vi "Stoerungen (65-128)- Allgemein.vi"(8 "Fehler (Eingang)":errorcluster caption="Fehler (Eingang, kein Fehler)") -> (0 "Fehler (Ausgang)":errorcluster)   [LabVIEW 2020, in "Stoermeldungen.lvlib"]
uses:
  Stoermeldungen.lvlib
  Stoerungen 65-128.ctl
  Seiten/Anlagengrenzwerte/Anlagen-Parameternamen.ctl
  Aktion Anlagengrenzen pruefen.ctl
  FGV Stoerungen Aktionen.ctl
  Verwaltung/FGV IN Aktionen.ctl
  Verwaltung/FGV OUT Aktionen.ctl
  Allgemein/FGV Analysator aktiv.ctl
  Konfig-Dateien/FGV Betriebsdaten Aktionen.ctl
  Allgemein/FGV Zustaende Aktionen.ctl
  Funktionstasten/Zustaende.ctl
  Stickstoff Befuellung/Aktionen Stockstoff Befuellung.ctl
  Seiten/Anlagengrenzwerte/Anlagengrenzwerte.lvlib
  Stickstoff Befuellung/Stickstoff Befuellung.lvlib
  Verwaltung/Verwaltung - cRIO.lvlib
  Allgemein/Allgemein.lvlib
  Konfig-Dateien/Konfig-Dateien.lvlib
  Funktionstasten/Funktionstasten.lvlib
  Externe Stickstoff Befuellung/Externe Stickstoff Befuellung.lvlib
  Externe Stickstoff Befuellung/Aktionen Externe Stockstoff Befuellung.ctl
panel:
  # "Störmeldungen:\n\nAllgemein (65-128)"
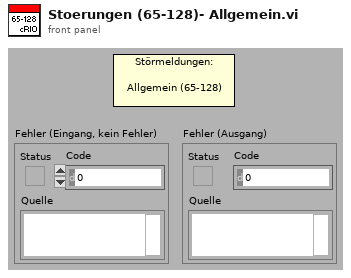
[diagram p1: front panel]
types:
  T1 = typedef "Funktionstasten.lvlib/Zustaende.ctl" = enum16{"Standby", "Pause", "Eco", "Messen", "Kalibrieren", "Spülen Filter", "Spülen Leitung", "Umgebungsluft", "0-Gas", "Cal-Gas", "CG zu PNS", "-------------", "Init 1", "Init 2", "Init 3", "Init 4", "Messen vorbereiten", "Messen durchführen", "Exit"}
  T2 = typedef "Allgemein.lvlib/FGV Zustaende Aktionen.ctl" = enum16{"lesen", "Zustand PC", "Zustand cRIO", "Bildnummer", "Samplepoint", "Sysloglevel"}
  T3 = typedef "Konfig-Dateien.lvlib/FGV Betriebsdaten Aktionen.ctl" = enum16{"lesen", "Anlagengrenzw.", "PID Param.", "Sonstige", "Sensor Para."}
  T4 = typedef "Allgemein.lvlib/FGV Analysator aktiv.ctl" = enum16{"lesen", "Analysator", "CG Aufschaltung", "KAL Zustand", "AutaKal GT?"}
  T5 = typedef "Verwaltung - cRIO.lvlib/FGV OUT Aktionen.ctl" = enum16{"lesen", "ANA OUT", "DO 0-31", "DO 32-47"}
  T6 = typedef "Verwaltung - cRIO.lvlib/FGV IN Aktionen.ctl" = enum16{"lesen", "DI", "AI", "Fühler Br.", "TC", "Fühler Br. TC"}
  T7 = typedef "Stoermeldungen.lvlib/FGV Stoerungen Aktionen.ctl" = enum16{"lesen", "Störung aktiv?", "1-64", "65-128"}
  T8 = typedef "Stoermeldungen.lvlib/Aktion Anlagengrenzen pruefen.ctl" = enum16{"Temp.", "HKL", "Druck", "SS Temp."}
  T9 = typedef "Anlagengrenzwerte.lvlib/Anlagen-Parameternamen.ctl" = enum16{"Eingangsdruck FT-IR:", "Durchfluss FT-IR:", "Durchfluss CalGas", "Druck Ausgang", "Druck Kalter Block", "Heizleitung intern", "Heizleitung zu FT-IR", "Heizung Filter:", "Heizung Pumpe:", "HL Extern SP1", "HL Extern SP2", "FT-IR Messzelle", "Schaltschrank", "Gaskühler"}
  T10 = typedef "Stoermeldungen.lvlib/Stoerungen 65-128.ctl" = cluster{"ERR. 65":bool, "ERR. 66":bool, "ERR. 67":bool, "ERR. 68":bool, "ERR. 69":bool, "ERR. 70":bool, "ERR. 71":bool, "ERR. 72":bool, "ERR. 73":bool, "ERR. 74":bool, "ERR. 75":bool, "ERR. 76":bool, "ERR. 77":bool, "ERR. 78":bool, "ERR. 79":bool, "ERR. 80":bool, "ERR. 81":bool, "ERR. 82":bool, "ERR. 83":bool, "ERR. 84":bool, "ERR. 85":bool, "ERR. 86":bool, "ERR. 87":bool, "ERR. 88":bool, "ERR. 89":bool, "ERR. 90":bool, "ERR. 91":bool, "ERR. 92":bool, "ERR. 93":bool, "ERR. 94":bool, "ERR. 95":bool, "ERR. 96":bool, "ERR. 97":bool, "ERR. 98":bool, "ERR. 99":bool, "ERR. 100":bool, "ERR. 101":bool, "ERR. 102":bool, "ERR. 103":bool, "ERR. 104":bool, "ERR. 105":bool, "ERR. 106":bool, "ERR. 107":bool, "ERR. 108":bool, "ERR. 109":bool, "ERR. 110":bool, "ERR. 111":bool, "ERR. 112":bool, "ERR. 113":bool, "ERR. 114":bool, "ERR. 115":bool, "ERR. 116":bool, "ERR. 117":bool, "ERR. 118":bool, "ERR. 119":bool, "ERR. 120":bool, "ERR. 121":bool, "ERR. 122":bool, "ERR. 123":bool, "ERR. 124":bool, "ERR. 125":bool, "ERR. 126":bool, "ERR. 127":bool, "ERR. 128":bool}
  T11 = typedef "Verwaltung - cRIO.lvlib/Digital Ausgaenge 32-63.ctl" = cluster{"O32: Messgaspumpe EIN":bool, "O33: (Umgebungsluftpumpe)":bool, "O34: (Kondensatpumpe GK)":bool, "O35: Klima/Lüfter EIN":bool, "O36: Versorgung Heizungen":bool, "O37: Versorgung Heizungen":bool, "O38: (Gaskühler EIN (Freigabe))":bool, "O39: Störung FAS LP":bool, "O40: (Heizung Filterblock)":bool, "O41: Heizung HL zu FT-IR":bool, "O42: Heizung HL Extern SP1":bool, "O43: Heizung HL Extern SP2":bool, "O44: Heizung Reserve":bool, "O45: Heizung Reserve":bool, "O46: Statusbeleuchtung grün":bool, "O47: Statusbeleuchtung rot":bool}
  T12 = typedef "Verwaltung - cRIO.lvlib/Digital Ausgaenge 0-31.ctl" = cluster{"O0: Druckluft Versorgung":bool, "O1: CG 1 (FB Eingang 1)":bool, "O2: CG 2 (Kühlung FT-IR EIN)":bool, "O3: CG 3 (FB Bypass)":bool, "O4: CG 4 (FB CalGas)":bool, "O5: CG 5 (FB spülen/UL)":bool, "O6: CG 6 (FB zum FT-IR)":bool, "O7: CG 7 (FB zum FID)":bool, "O8: CG 8 (FB Reserve)":bool, "O9: (FB Reserve)":bool, "O10: (FB Umgebungsluft FID)":bool, "O11: (FB zum Gaskühler)":bool, "O12: FB Stickstoff zu FT-IR":bool, "O13: Optikbox FT-IR spülen":bool, "O14: (Purifier deaktivieren)":bool, "O15: (Umschaltung Purifier/Stickstoff)":bool, "O16: N2 Einblasung":bool, "O17: LSP LN2 Nachfüllung":bool, "O18: (Reserve)":bool, "O19: (Pumpe Eingang1)":bool, "O20: (Pumpe Eingang2)":bool, "O21: (Pumpe Spülen1)":bool, "O22: (Pumpe Spülen2)":bool, "O23: (Reserve)":bool, "O24: CalGas 1":bool, "O25: CalGas 2":bool, "O26: CG 3-8 (CalGas 3)":bool, "O27: Stickstoff aufschalten":bool, "O28: CG zu PNS":bool, "O29: FTIR Standby Spülung":bool, "O30: CG zu Entnahme(T90)":bool, "O31: (Purifier regenerieren)":bool}
  T13 = typedef "Status Analysatoren.lvlib/Status Analysatoren_Anzeige.ctl" = cluster{"FT-IR":bool, "FID":bool, "PMA":bool}
  T14 = typedef "Verwaltung - cRIO.lvlib/Digital Eingaenge 0-15.ctl" = cluster{"I0: N2 Nachf. FT-IR voll":bool, "I1: N2 Nachf. Vorrat leer":bool, "I2: (Klimaanlage eingeschaltet)":bool, "I3: (Klimaanlage Störung)":bool, "I4: Trigger Eingang (Messdaten sp.)":bool, "I5: Reserve":bool, "I6: Reserve":bool, "I7: Reserve":bool, "I8: Druckschalter Versorgung ok":bool, "I9: Reserve":bool, "I10: Reserve":bool, "I11: Reserve":bool, "I12: Drucksch. N2 Versorgung":bool, "I13: Reserve":bool, "I14: Drucksch. N2 Optikbox":bool, "I15: (Füllstand Kondensatbehälter)":bool}
  T15 = typedef "Verwaltung - cRIO.lvlib/Analog Eingaenge.ctl" = cluster{"AI0: Durchfluss FT-IR":sgl, "AI1: Druck Ausgang":sgl, "AI2: Umgebungsdruck":sgl, "AI3: Druck FT-IR":sgl, "AI4: Druck CalGas":sgl, "AI5: Reserve":sgl, "AI6: Reserve":sgl, "AI7: Reserve":sgl, "Rohwert Durchfluss FT-IR":sgl, "Rohwert Druck Ausgang":sgl, "Rohwert Umgebungsdruck":sgl, "Rohwert Druck FT-IR":sgl, "Rohwert Druck CalGas":sgl, "Rohwert AI5":sgl, "Rohwert AI6":sgl, "Rohwert AI7":sgl, "Rohwert Diffdruck mbar FTIR":sgl}
  T16 = typedef "Verwaltung - cRIO.lvlib/TC Eingaenge.ctl" = cluster{"TC0: Reserve":sgl, "TC1: HL zu FT-IR":sgl, "TC2: HL Extern SP1":sgl, "TC3: HL Extern SP2":sgl, "TC4: Reserve":sgl, "TC5: Reserve":sgl, "TC6: Reserve":sgl, "TC7: Reserve":sgl, "TC8: FT-IR":sgl, "TC9: Reserve":sgl, "TC10: Schaltschrank":sgl, "TC11: Umgebung":sgl}
  T17 = typedef "Verwaltung - cRIO.lvlib/Fuehler Bruch AI.ctl" = cluster{"AI0: Durchfluss FT-IR":bool, "AI1: Druck Ausgang":bool, "AI2: Umgebungsdruck":bool, "AI3: Druck FT-IR":bool, "AI4: Druck CalGas":bool, "AI5: Reserve":bool, "AI6: Reserve":bool, "AI7: Reserve":bool}
  T18 = typedef "Stickstoff Befuellung.lvlib/Aktionen Stockstoff Befuellung.ctl" = enum16{"lesen", "Befüllen vorbereiten", "Befüllen", "Befüllen beenden", "Warten", "deaktiviert", "initialisieren", "anstehender Fehler"}
  T19 = typedef "Externe Stickstoff Befuellung.lvlib/Aktionen Externe Stockstoff Befuellung.ctl" = enum16{"lesen", "Befüllen vorbereiten", "Befüllen", "Befüllen beenden", "Warten", "deaktiviert", "initialisieren"}
  T20 = typedef "Erweiterte Konfig.lvlib/Sonstige Parameter.ctl" = cluster{"Lüfter langsam":sgl, "Lüfter schnell":sgl, "FT-IR Kühlung Soll":sgl, "FT-IR Kühlung Max":sgl, "Überwachung":T21, "Befüllung aktiv":T22, "Stickstoff Befüllzeit":sgl, "Befüllintervall":sgl, "Kalibrierwert FT-IR":sgl, "Offset Ausgang":sgl, "Offset FT-IR":sgl, "Offset Druck FT-IR":sgl, "Dichtheitstest Zeit":sgl, "Dichtheitstest Abfall":sgl, "Dichtheitstest Umfang":T23, "Offset Umgebung":sgl, "Max Taupunkt":sgl, "Pumpendrehzahl":sgl, "ext. Befüllung":T22, "Ext. Stickstoff Befüllzeit":sgl}
  T21 = typedef "Auswahlfeld.ctl" = u16
  T22 = typedef "LogKonfig.lvlib/Auswahlfeld aktiviert-deaktiviert.ctl" = u16
  T23 = typedef "Erweiterte Konfig.lvlib/Dichtheitstest Umfang.ctl" = u16
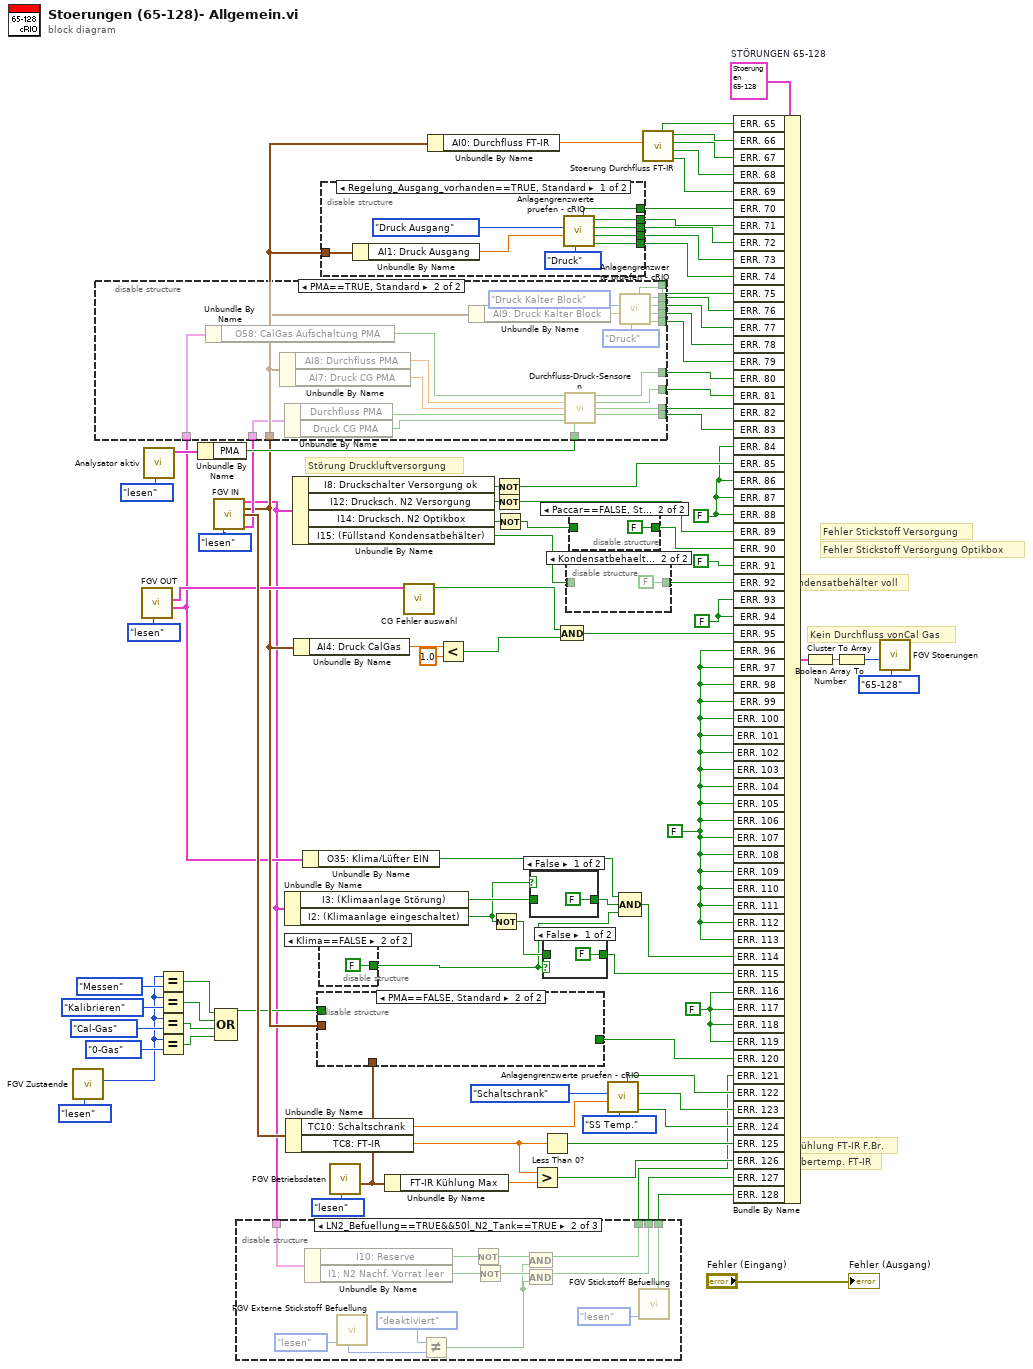
[diagram p0: block diagram]
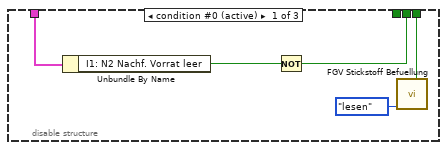
[diagram p3: hidden frame]
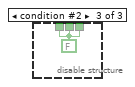
[diagram p4: hidden frame]
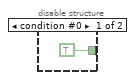
[diagram p7: hidden frame]
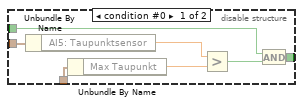
[diagram p9: hidden frame]
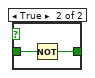
[diagram p10: hidden frame]
diagram:
  w41 = FALSE ("ERR. 86")
  w29 = FALSE ("ERR. 102")
  w33 = FALSE ("ERR. 102")
  w74 = FALSE ("ERR. 99")
  w90 = T10 {"ERR. 65"=FALSE, "ERR. 66"=FALSE, "ERR. 67"=FALSE, "ERR. 68"=FALSE, "ERR. 69"=FALSE, "ERR. 70"=FALSE, "ERR. 71"=FALSE, "ERR. 72"=FALSE, "ERR. 73"=FALSE, "ERR. 74"=FALSE, "ERR. 75"=FALSE, "ERR. 76"=FALSE, "ERR. 77"=FALSE, "ERR. 78"=FALSE, "ERR. 79"=FALSE, "ERR. 80"=FALSE, "ERR. 81"=FALSE, "ERR. 82"=FALSE, "ERR. 83"=FALSE, "ERR. 84"=FALSE, "ERR. 85"=FALSE, "ERR. 86"=FALSE, "ERR. 87"=FALSE, "ERR. 88"=FALSE, "ERR. 89"=FALSE, "ERR. 90"=FALSE, "ERR. 91"=FALSE, "ERR. 92"=FALSE, "ERR. 93"=FALSE, "ERR. 94"=FALSE, "ERR. 95"=FALSE, "ERR. 96"=FALSE, "ERR. 97"=FALSE, "ERR. 98"=FALSE, "ERR. 99"=FALSE, "ERR. 100"=FALSE, "ERR. 101"=FALSE, "ERR. 102"=FALSE, "ERR. 103"=FALSE, "ERR. 104"=FALSE, "ERR. 105"=FALSE, "ERR. 106"=FALSE, "ERR. 107"=FALSE, "ERR. 108"=FALSE, "ERR. 109"=FALSE, "ERR. 110"=FALSE, "ERR. 111"=FALSE, "ERR. 112"=FALSE, "ERR. 113"=FALSE, "ERR. 114"=FALSE, "ERR. 115"=FALSE, "ERR. 116"=FALSE, "ERR. 117"=FALSE, "ERR. 118"=FALSE, "ERR. 119"=FALSE, "ERR. 120"=FALSE, "ERR. 121"=FALSE, "ERR. 122"=FALSE, "ERR. 123"=FALSE, "ERR. 124"=FALSE, "ERR. 125"=FALSE, "ERR. 126"=FALSE, "ERR. 127"=FALSE, "ERR. 128"=FALSE}  # STÖRUNGEN 65-128
  # "Fehler Stickstoff Versorgung Optikbox"
  # "Übertemp. FT-IR"
  # "Kühlung FT-IR F.Br."
  # "Kondensatbehälter voll"
  # "Störung Druckluftversorgung"
  # "Kein Durchfluss vonCal Gas"
  # "Fehler Stickstoff Versorgung"
  n1 = call "FGV Zustaende.vi"("Aktionen"=FGV_Zustaende_Aktionen."lesen") -> ("Zustand cRIO"=w17:T1)  [unwired: 6 in, 4 out]
  n2 = call "FGV OUT.vi"("Aktion"=FGV_OUT_Aktionen."lesen") -> ("DO 32-63"=w14:T11, "DO 0-31"=w50:T12)  [unwired: 7 in, 2 out]
  n3 = call "Analysator aktiv.vi"("Aktion"=FGV_Analysator_aktiv."lesen") -> ("Status Analysatoren"=w48:T13)  [unwired: 7 in, 3 out]
  n4 = Equal?(x=w17, y=Zustaende."Messen" ("Zustand PC")) -> (x = y?=w28:bool)
  n5 = Equal?(x=w17, y=Zustaende."Kalibrieren" ("Zustand PC")) -> (x = y?=w27:bool)
  n6 = Equal?(x=w17, y=Zustaende."Cal-Gas" ("Zustand PC")) -> (x = y?=w26:bool)
  n7 = Equal?(x=w17, y=Zustaende."0-Gas" ("Zustand PC")) -> (x = y?=w25:bool)
  n8 = Unbundle By Name(w48) -> ("PMA"=w47:bool)
  n9 = call "FGV IN.vi"("Aktion"=FGV_IN_Aktionen."lesen") -> ("DI"=w11:T14, "Analog Eingänge"=w30:T15, "TC Eingänge"=w64:T16, "Fühler Bruch AI"=w46:T17)  [unwired: 10 in, 1 out]
  n10 = disable-structure shown="PMA==TRUE, Standard" {
    disable-tunnel: [_ w112] -> w55
    disable-tunnel: [_ w111] -> w54
    disable-tunnel: [_ w110] -> w53
    disable-tunnel: [_ w109] -> w52
    disable-tunnel: [_ w108] -> w51
    disable-tunnel: w47 -> [_ w107]
    disable-tunnel: w46 -> [_ w106]
    disable-tunnel: [_ w100] -> w45
    disable-tunnel: [_ w99] -> w44
    disable-tunnel: [_ w98] -> w43
    disable-tunnel: [_ w97] -> w42
    disable-tunnel: w30 -> [_ w96]
    disable-tunnel: w14 -> [_ w95]
    frame condition #0 (active) {
    }
    frame condition #1 {
      n11 = Unbundle By Name(w95) -> ("O58: CalGas Aufschaltung PMA"=w103:bool)
      n12 = Unbundle By Name(w96) -> ("AI8: Durchfluss PMA"=w102:sgl, "AI7: Druck CG PMA"=w101:sgl)
      n13 = Unbundle By Name(w106) -> ("Durchfluss PMA"=w104:bool, "Druck CG PMA"=w105:bool)
      n14 = Unbundle By Name(w96) -> ("AI9: Druck Kalter Block"=w92:sgl)
      n15 = call "Durchfluss-Druck-Sensoren.vi"("CalGas Ventil"=w103, "Istwert Durchfluss"=w102, "Istwert Druck"=w101, "F.Bruch Durchfluss"=w104, "F.Bruch Druck"=w105, "Analysator aktiv?"=w107) -> ("Fühlerbruch Durchflusssensor"=w100:bool, "Durchfluss"=w99:bool, "Fühlerbruch Drucksensor"=w98:bool, "Druck CalGas"=w97:bool)  [unwired: 6 in]
      n16 = call "Anlagengrenzwerte pruefen - cRIO.vi"("Aktion"=Aktion_Anlagengrenzen_pruefen."Druck", "Wert"=w92, "Anlagen-Parametername"=Anlagen-Parameternamen."Druck Kalter Block") -> ("AbschMax"=w108:bool, "AbschMin"=w109:bool, "WarnMax"=w110:bool, "WarnMin"=w111:bool, "F.Br."=w112:bool)  [unwired: 4 in]
    }
  }
  n17 = Compound Arithmetic op=OR(w28, w27, w26, w25) -> (w18:bool)
  n18 = disable-structure shown="LN2_Befuellung==TRUE&&50l_N2_Tank==TRUE" {
    disable-tunnel: [w116 w129 w131] -> w40
    disable-tunnel: [w114 w120 w131] -> w39
    disable-tunnel: w11 -> [w113 w126 _]
    disable-tunnel: [_ w119 w131] -> w1
    frame condition #0 (active) {
      n19 = Unbundle By Name(w113) -> ("I1: N2 Nachf. Vorrat leer"=w115:bool)
      n20 = Not(x=w115) -> (.not. x?=w114:bool)
      n21 = call "FGV Stickstoff Befuellung.vi"("Aktion"=Aktionen_Stockstoff_Befuellung."lesen") -> ("Timeout"=w116:bool)  [unwired: 4 in, 6 out]
    }
    frame condition #1 {
      n22 = Unbundle By Name(w126) -> ("I10: Reserve"=w122:bool, "I1: N2 Nachf. Vorrat leer"=w128:bool)
      n23 = call "FGV Externe Stickstoff Befuellung.vi"("Aktion"=Aktionen_Externe_Stockstoff_Befuellung."lesen") -> ("Aktion"=w125:T19)  [unwired: 4 in, 6 out]
      n24 = Not Equal?(x=Aktionen_Externe_Stockstoff_Befuellung."deaktiviert", y=w125) -> (x != y?=w118:bool)
      n25 = Not(x=w122) -> (.not. x?=w121:bool)
      n26 = Not(x=w128) -> (.not. x?=w127:bool)
      n27 = And(x=w121, y=w118) -> (x .and. y?=w119:bool)
      n28 = And(x=w127, y=w118) -> (x .and. y?=w120:bool)
      n29 = call "FGV Stickstoff Befuellung.vi"("Aktion"=Aktionen_Stockstoff_Befuellung."lesen") -> ("Timeout"=w129:bool)  [unwired: 4 in, 6 out]
    }
    frame condition #2 {
      w131 = FALSE
    }
  }
  n30 = Unbundle By Name(w11) -> ("I3: (Klimaanlage Störung)"=w10:bool, "I2: (Klimaanlage eingeschaltet)"=w9:bool)
  n31 = Unbundle By Name(w64) -> ("TC10: Schaltschrank"=w63:sgl, "TC8: FT-IR"=w62:sgl)
  n32 = Unbundle By Name(w11) -> ("I8: Druckschalter Versorgung ok"=w89:bool, "I12: Drucksch. N2 Versorgung"=w84:bool, "I14: Drucksch. N2 Optikbox"=w4:bool, "I15: (Füllstand Kondensatbehälter)"=w5:bool)
  n33 = Unbundle By Name(w30) -> ("AI4: Druck CalGas"=w83:sgl)
  n34 = Unbundle By Name(w14) -> ("O35: Klima/Lüfter EIN"=w13:bool)
  n35 = disable-structure shown="Klima==FALSE" {
    disable-tunnel: [TRUE ("Klimaanlage vorhanden") FALSE ("Klimaanlage vorhanden")] -> w7
    frame condition #0 {
    }
    frame condition #1 (active) {
    }
  }
  n36 = disable-structure shown="Regelung_Ausgang_vorhanden==TRUE, Standard" {
    disable-tunnel: [w140 _] -> w80
    disable-tunnel: [w139 _] -> w79
    disable-tunnel: [w138 _] -> w78
    disable-tunnel: [w137 _] -> w77
    disable-tunnel: [w136 _] -> w76
    disable-tunnel: w30 -> [w134 _]
    frame condition #0 (active) {
      n37 = Unbundle By Name(w134) -> ("AI1: Druck Ausgang"=w142:sgl)
      n38 = call "Anlagengrenzwerte pruefen - cRIO.vi"("Aktion"=Aktion_Anlagengrenzen_pruefen."Druck", "Wert"=w142, "Anlagen-Parametername"=Anlagen-Parameternamen."Druck Ausgang") -> ("AbschMax"=w136:bool, "AbschMin"=w137:bool, "WarnMax"=w138:bool, "WarnMin"=w139:bool, "F.Br."=w140:bool)  [unwired: 4 in]
    }
    frame condition #1 {
    }
  }
  n39 = call "FGV Betriebsdaten.vi"("Aktionen"=FGV_Betriebsdaten_Aktionen."lesen") -> ("Sonstige"=w31:T20)  [unwired: 7 in, 3 out]
  n40 = disable-structure shown="PMA==FALSE, Standard" {
    disable-tunnel: w31 -> [w149 _]
    disable-tunnel: w30 -> [w147 _]
    disable-tunnel: [w144 _] -> w19
    disable-tunnel: w18 -> [w143 _]
    frame condition #0 {
      n41 = Unbundle By Name(w147) -> ("AI5: Taupunktsensor"=w146:sgl)
      n42 = Unbundle By Name(w149) -> ("Max Taupunkt"=w148:sgl)
      n43 = Greater?(x=w146, y=w148) -> (0:w145:bool)
      n44 = And(x=w143, y=w145) -> (x .and. y?=w144:bool)
    }
    frame condition #1 (active) {
    }
  }
  n45 = Unbundle By Name(w31) -> ("FT-IR Kühlung Max"=w65:sgl)
  n46 = call "CG Fehler auswahl.vi"("DO 0-31"=w50) -> ("Boolesch"=w71:bool)  [unwired: 10 in]
  n47 = Unbundle By Name(w30) -> ("AI0: Durchfluss FT-IR"=w56:sgl)
  n48 = Less?(x=w83, y=sgl 1.0) -> (x < y?=w81:bool)
  n49 = Not(x=w9) -> (.not. x?=w15:bool)
  n50 = Not(x=w89) -> (.not. x?=w73:bool)
  n51 = Not(x=w84) -> (.not. x?=w70:bool)
  n52 = Not(x=w4) -> (.not. x?=w3:bool)
  n53 = case shown="False" w9 {
    tunnel: w10 -> [_ w152]
    tunnel: [FALSE w151] -> w16
    frame False {
    }
    frame True {
      n54 = Not(x=w152) -> (.not. x?=w151:bool)
    }
  }
  n55 = Greater?(x=w62, y=w65) -> (0:w38:bool)
  n56 = Less Than 0?(x=w62) -> (x < 0?=w37:bool)
  n57 = case shown="False" w7 {
    tunnel: w15 -> [_ w154]
    tunnel: [FALSE w154] -> w8
    frame False {
    }
    frame True {
    }
  }
  n58 = And(x=w71, y=w81) -> (x .and. y?=w75:bool)
  n59 = disable-structure shown="Kondensatbehaelter==FALSE" {
    disable-tunnel: [w155 FALSE ("I15: (Füllstand Kondensatbehälter)")] -> w6
    disable-tunnel: w5 -> [w155 _]
    frame condition #0 (active) {
    }
    frame condition #1 {
    }
  }
  n60 = disable-structure shown="Paccar==FALSE, Standard" {
    disable-tunnel: w3 -> [w157 _]
    disable-tunnel: [w157 FALSE] -> w2
    frame condition #0 {
    }
    frame condition #1 (active) {
    }
  }
  n61 = call "Anlagengrenzwerte pruefen - cRIO.vi"("Aktion"=Aktion_Anlagengrenzen_pruefen."SS Temp.", "Wert"=w63, "Anlagen-Parametername"=Anlagen-Parameternamen."Schaltschrank") -> ("AbschMax"=w34:bool, "WarnMax"=w35:bool, "F.Br."=w36:bool)  [unwired: 4 in, 2 out]
  n62 = Compound Arithmetic op=AND ("Mehrfacharithmetik")(w13, w16, w7) -> (w12:bool)
  n63 = call "Stoerung Durchfluss FT-IR.vi"("Durchfluss FT-IR"=w56) -> ("AbschMax"=w57:bool, "AbschMin"=w58:bool, "WarnMax"=w59:bool, "WarnMin"=w60:bool, "F.Br."=w61:bool)  [unwired: 6 in]
  n64 = Bundle By Name(cluster=w90, "ERR. 65"=w61, "ERR. 66"=w60, "ERR. 67"=w59, "ERR. 68"=w58, "ERR. 69"=w57, "ERR. 70"=w80, "ERR. 71"=w79, "ERR. 72"=w78, "ERR. 73"=w77, "ERR. 74"=w76, "ERR. 75"=w55, "ERR. 76"=w54, "ERR. 77"=w53, "ERR. 78"=w52, "ERR. 79"=w51, "ERR. 80"=w45, "ERR. 81"=w44, "ERR. 82"=w43, "ERR. 83"=w42, "ERR. 84"=w41, "ERR. 85"=w73, "ERR. 86"=w41, "ERR. 87"=w41, "ERR. 88"=w41, "ERR. 89"=w70, "ERR. 90"=w2, "ERR. 91"=FALSE ("ERR. 90"), "ERR. 92"=w6, "ERR. 93"=w74, "ERR. 94"=w74, "ERR. 95"=w75, "ERR. 96"=w33, "ERR. 97"=w33, "ERR. 98"=w33, "ERR. 99"=w33, "ERR. 100"=w33, "ERR. 101"=w33, "ERR. 102"=w33, "ERR. 103"=w33, "ERR. 104"=w33, "ERR. 105"=w33, "ERR. 106"=w33, "ERR. 107"=w33, "ERR. 108"=w33, "ERR. 109"=w33, "ERR. 110"=w33, "ERR. 111"=w33, "ERR. 112"=w33, "ERR. 113"=w33, "ERR. 114"=w12, "ERR. 115"=w8, "ERR. 116"=w29, "ERR. 117"=w29, "ERR. 118"=w29, "ERR. 119"=w29, "ERR. 120"=w19, "ERR. 121"=w1, "ERR. 122"=w36, "ERR. 123"=w35, "ERR. 124"=w34, "ERR. 125"=w37, "ERR. 126"=w38, "ERR. 127"=w39, "ERR. 128"=w40) -> (w87:T10)
  n65 = Cluster To Array(cluster=w87) -> (array=w86:bool[])
  n66 = Boolean Array To Number ("Boolesches Array nach Zahl")(Boolean array=w86) -> (number=w68:u64)
  n67 = call "FGV Stoerungen.vi"("Aktionen"=FGV_Stoerungen_Aktionen."65-128", "65-128"=w68) -> ()  [unwired: 7 in, 3 out]
  "Fehler (Ausgang)" <- "Fehler (Eingang)"
